vi "Write Reference amplitude.vi"(8 "error in (no error)":errorcluster, 10 "Reference amplitude":dbl, 11 "Lock-in Detector in":refnum<class "Lock-in Detector.lvclass">) -> (0 "error out":errorcluster, 3 "Lock-in Detector out":refnum<class "Lock-in Detector.lvclass">)   [LabVIEW 2020, in "Lock-in Detector.lvclass"]
uses:
  Lock-in Detector.lvclass
  Lock-in Detector.lvclass/Lock-in Detector.ctl
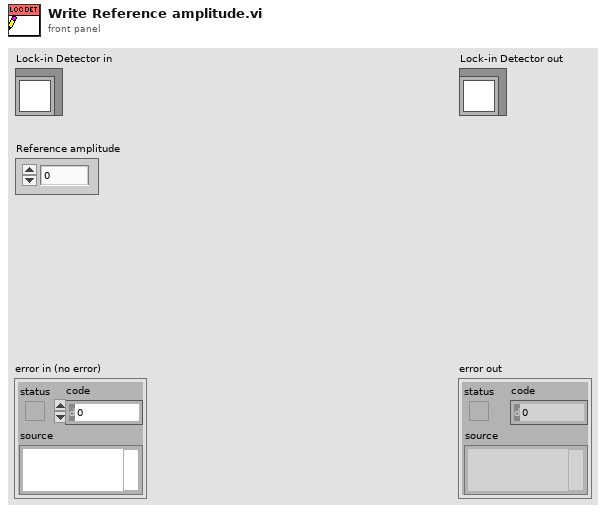
[diagram p1: front panel]
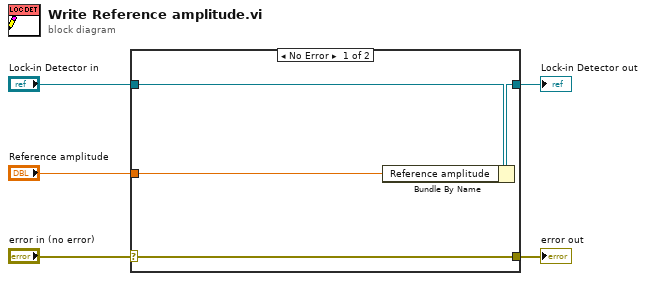
[diagram p0: block diagram]
diagram:
  n1 = case shown="No Error" "error in (no error)" {
    selector: "error in (no error)" -> [w9 w10]
    tunnel: [w9 w10] -> w4
    tunnel: [w7 w11] -> w2
    tunnel: "Lock-in Detector in" -> [w8 w11]
    tunnel: "Reference amplitude" -> [w6 _]
    frame No Error {
      n2 = Bundle By Name(cluster=w8, "Reference amplitude"=w6) -> (w7:refnum<class "Lock-in Detector.lvclass">)
    }
    frame Error {
    }
  }
  "error out" <- w4
  "Lock-in Detector out" <- w2
